vi "detChildElementByName.vi"(8 "error in (no error)":errorcluster, 10 "childName":string, 11 "Element in":refnum<class "XMLParser.lvclass">) -> (0 "error out":errorcluster, 1 "childAttributes":T1[](array[typedef]), 2 "childXML":string, 3 "Element out":refnum<class "XMLParser.lvclass">)   [LabVIEW 2016, in "XML.lvlib" / "XMLParser.lvclass"]
doc: "This method parses the child contents based on the input parameter, and handles attributes as necessary."
uses:
  <userlib>/Common/XML/XMLParser/XMLParser.lvclass
  <userlib>/Common/XML/Typedefs/AttributeElements.ctl
  <userlib>/Common/XML/XMLParser/XMLParser.lvclass/XMLParser.ctl
  <userlib>/Common/XML/XMLAttributeParser/XMLAttributeParser.lvclass
  <userlib>/Common/XML/XML.lvlib
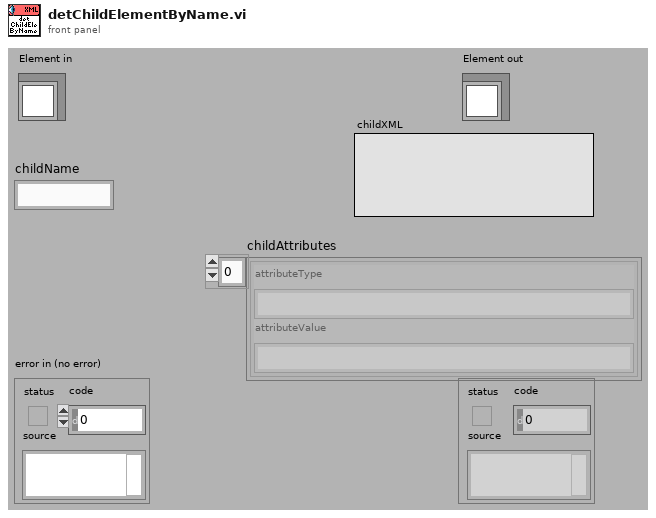
[diagram p1: front panel]
types:
  T1 = typedef "XML.lvlib/AttributeElements.ctl" = cluster{"attributeType":string, "attributeValue":string}
  T2 = cluster{"result string":string, "result string":string}[]
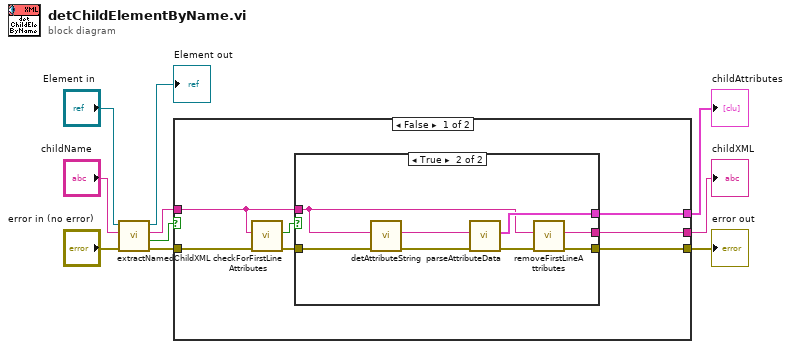
[diagram p0: block diagram]
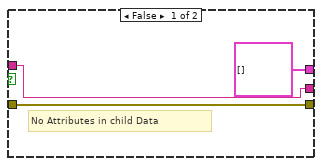
[diagram p2: hidden frame]
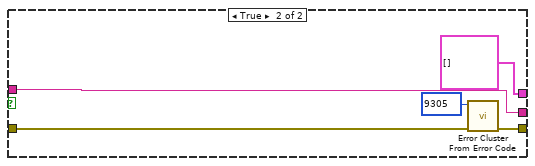
[diagram p3: hidden frame]
diagram:
  n1 = call <userlib>:"extractNamedChildXML.vi"("error in (no error)"="error in (no error)", "childName"="childName", "ReadElement in"="Element in") -> ("error out"=w7:errorcluster, "ChildContentsEmpty"=w8:bool, "childXML"=w6:string, "ReadElement out"=→"Element out":refnum<class "XMLParser.lvclass">)  [unwired: 5 in]
  n2 = case shown="False" w8 {
    tunnel: w7 -> [w17 w33]
    tunnel: [w11 w32] -> w2
    tunnel: w6 -> [w15 w29]
    tunnel: [w13 T2 [] ("attributeData")] -> w4
    tunnel: [w12 w29] -> w3
    frame False {
      n3 = call <userlib>:"checkForFirstLineAttributes.vi"("error in (no error)"=w17, "XML In"=w15) -> ("error out"=w14:errorcluster, "firstLineAttributeFound"=w16:bool)  [unwired: 7 in, 1 out]
      n4 = case shown="True" w16 {
        tunnel: w14 -> [w19 w28]
        tunnel: [w19 w21] -> w11
        tunnel: [w18 w22] -> w12
        tunnel: [T2 [] ("attributeData") w26] -> w13
        tunnel: w15 -> [w18 w23]
        frame False {
          # "No Attributes in child Data"
        }
        frame True {
          n5 = call <userlib>:"detAttributeString.vi"("error in (no error)"=w28, "XML In"=w23) -> ("error out"=w27:errorcluster, "AttributeString"=w25:string)  [unwired: 6 in, 2 out]
          n6 = call <userlib>:"parseAttributeData.vi"("error in (no error)"=w27, "XMLString in"=w25) -> ("error out"=w24:errorcluster, "attributeData"=w26:T2)  [unwired: 7 in, 1 out]
          n7 = call <userlib>:"removeFirstLineAttributes.vi"("error in (no error)"=w24, "XMLString in"=w23) -> ("error out"=w21:errorcluster, "XMLString out"=w22:string)  [unwired: 8 in]
        }
      }
    }
    frame True {
      n8 = call <vilib>:"Error Cluster From Error Code.vi"("error in (no error)"=w33, "error code (0)"=9305) -> ("error out"=w32:errorcluster)  [unwired: 7 in]
    }
  }
  "error out" <- w2
  "childXML" <- w3
  "childAttributes" <- w4
